vi "EventMachine.vi"() -> ()   [LabVIEW 2020]
panel:
  out "Data":i32
  in  "Events":T1
  in  "Event Data":T2
  in  "TEST":bool
  in  "INIT":bool
  in  "Stop":bool
  out "error out":errorcluster
  in  "error in":errorcluster
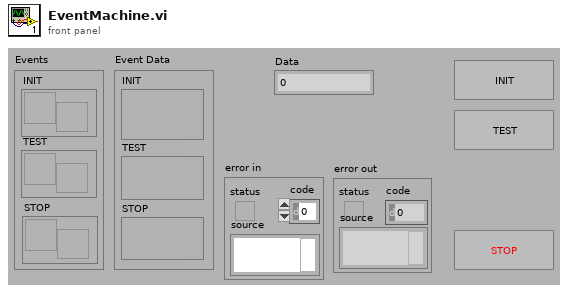
[diagram p1: front panel]
types:
  T1 = cluster{"INIT":refnum<user-event>, "TEST":refnum<user-event>, "STOP":refnum<user-event>}
  T2 = cluster{"INIT":variant, "TEST":variant, "STOP":variant}
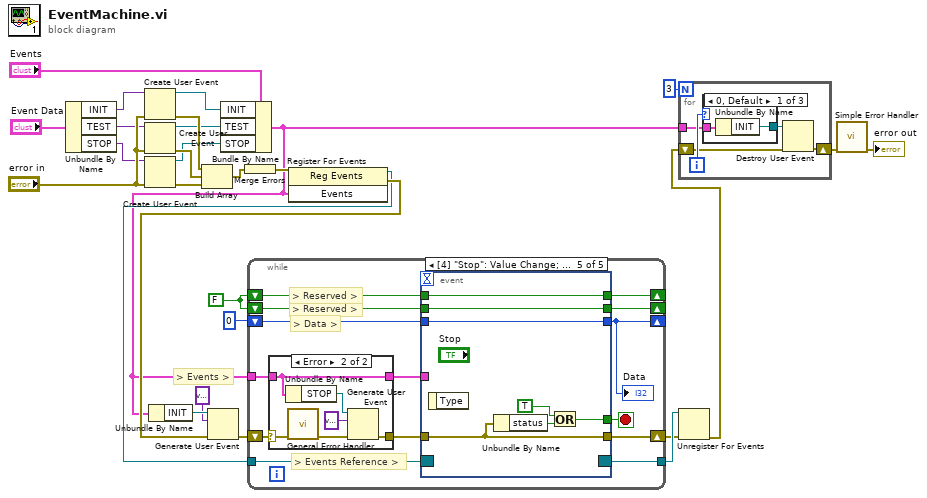
[diagram p0: block diagram]
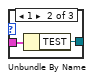
[diagram p2: hidden frame]
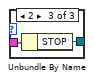
[diagram p3: hidden frame]
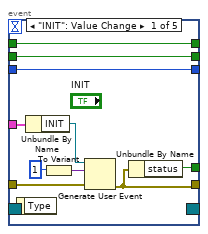
[diagram p4: hidden frame]
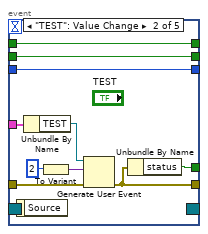
[diagram p5: hidden frame]
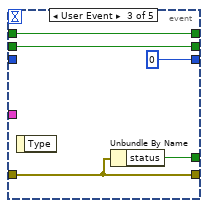
[diagram p6: hidden frame]
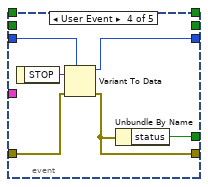
[diagram p7: hidden frame]
diagram:
  w19 = FALSE
  # "> Events >"
  n1 = Unbundle By Name("Event Data") -> ("INIT"=w12:variant, "TEST"=w11:variant, "STOP"=w6:variant)
  n2 = Create User Event(user event datatype=w12, error in="error in") -> (user event=w9:refnum<user-event>, error out=w17:errorcluster)
  n3 = Create User Event(user event datatype=w11, error in="error in") -> (user event=w8:refnum<user-event>, error out=w16:errorcluster)
  n4 = Create User Event(user event datatype=w6, error in="error in") -> (user event=w5:refnum<user-event>, error out=w3:errorcluster)
  n5 = Build Array(w17, w16, w3) -> (w15:errorcluster[])
  n6 = Bundle By Name(cluster="Events", "INIT"=w9, "TEST"=w8, "STOP"=w5) -> (w4:T1)
  n7 = Unbundle By Name(w4) -> ("INIT"=w7:refnum<user-event>)
  n8 = Merge Errors(w15) -> (w14:errorcluster)
  n9 = register-events(error in=w14, w4) -> (reference out=w25:refnum<event-registration>, error out=w27:errorcluster)  [unwired: 1 in]
  n10 = Generate User Event(user event=w7, event data cluster=variant ("event data"), error in=w27) -> (error out=w26:errorcluster)  [unwired: 1 in, 1 out]
  n11 = while {
    shift-right: [w41] -> w23
    shift-left: w26 -> [w35]
    shift-right: [w38] -> _
    shift-left: w19 -> [w36]
    shift-right: [w40] -> _
    shift-left: w19 -> [w39]
    shift-right: [w29] -> _
    shift-left: 0 -> [w37]
    tunnel: w25 -> [w33]
    tunnel: [w32] -> w24
    tunnel: w4 -> [w30]
    stop <- w42 stop-if-true
    # "> Events Reference >"
    # "> Data >"
    # "> Reserved >"
    # "> Reserved >"
    n12 = case shown="Error" w35 {
      selector: w35 -> [w82 w88]
      tunnel: [w82 w86] -> w34
      tunnel: [w81 w84] -> w31
      tunnel: w30 -> [w81 w84]
      frame No Error {
      }
      frame Error {
        n13 = Unbundle By Name(w84) -> ("STOP"=w85:refnum<user-event>)
        n14 = call <vilib>:"General Error Handler.vi"("error in (no error)"=w88) -> ("error out"=w87:errorcluster)  [unwired: 10 in, 4 out]
        n15 = Generate User Event(user event=w85, event data cluster=variant ("event data"), error in=w87) -> (error out=w86:errorcluster)  [unwired: 1 in, 1 out]
      }
    }
    n16 = event shown="[4] \"Stop\": Value Change;  <Events.STOP>: User Event" {
      selector: w33 -> [_ _ _ _ _]
      dyn-events: [_ _ _ _ _] -> w32
      timeout: _ -> [_ _ _ _ _]
      tunnel: w34 -> [w52 w62 w64 w71 w77]
      tunnel: [w51 w61 w64 w70 w77] -> w41
      tunnel: [w50 w60 w67 w73 w76] -> w42
      tunnel: w36 -> [w45 w55 w66 _ w80]
      tunnel: w39 -> [w44 w54 w65 _ w79]
      tunnel: w37 -> [w43 w53 _ w69 w78]
      tunnel: [w45 w55 w66 _ w80] -> w38
      tunnel: [w44 w54 w65 _ w79] -> w40
      tunnel: [w43 w53 0 w68 w78] -> w29
      tunnel: w31 -> [w49 w59 _ _ _]
      event "INIT": Value Change {
        n17 = event-data() -> ()  [unwired: 1 in, 1 out]
        n18 = Unbundle By Name(w49) -> ("INIT"=w48:refnum<user-event>)
        n19 = To Variant(anything=1) -> (Variant=w47:variant)
        n20 = Generate User Event(user event=w48, event data cluster=w47, error in=w52) -> (error out=w51:errorcluster)  [unwired: 1 in, 1 out]
        n21 = Unbundle By Name(w51) -> ("status"=w50:bool)
      }
      event "TEST": Value Change {
        n22 = event-data() -> ()  [unwired: 1 in, 1 out]
        n23 = Unbundle By Name(w59) -> ("TEST"=w58:refnum<user-event>)
        n24 = To Variant(anything=2) -> (Variant=w56:variant)
        n25 = Generate User Event(user event=w58, event data cluster=w56, error in=w62) -> (error out=w61:errorcluster)  [unwired: 1 in, 1 out]
        n26 = Unbundle By Name(w61) -> ("status"=w60:bool)
      }
      event User Event {
        n27 = event-data() -> ()  [unwired: 1 in, 1 out]
        n28 = Unbundle By Name(w64) -> ("status"=w67:bool)
      }
      event User Event {
        n29 = event-data() -> ("STOP"=w72:variant)  [unwired: 1 in]
        n30 = Variant To Data(error in=w71, type=w69, Variant=w72) -> (data=w68:i32, error out=w70:errorcluster)
        n31 = Unbundle By Name(w70) -> ("status"=w73:bool)
      }
      event "Stop": Value Change; User Event {
        n32 = event-data() -> ()  [unwired: 1 in, 1 out]
        n33 = Unbundle By Name(w77) -> ("status"=w74:bool)
        n34 = Or(x=TRUE ("y"), y=w74) -> (x .or. y?=w76:bool)
      }
    }
    "Data" <- w29
  }
  n35 = Unregister For Events(event registration refnum=w24, error in=w23) -> (error out=w21:errorcluster)
  n36 = for {
    N: 3 -> [_]
    shift-right: [w91] -> w20
    shift-left: w21 -> [w92]
    tunnel: w4 -> [w90]
    i -> [w93]
    n37 = case shown="0, Default" w93 {
      tunnel: [w95 w97 w99] -> w89
      tunnel: w90 -> [w94 w96 w98]
      frame 0, Default {
        n38 = Unbundle By Name(w94) -> ("INIT"=w95:refnum<user-event>)
      }
      frame 1 {
        n39 = Unbundle By Name(w96) -> ("TEST"=w97:refnum<user-event>)
      }
      frame 2 {
        n40 = Unbundle By Name(w98) -> ("STOP"=w99:refnum<user-event>)
      }
    }
    n41 = Destroy User Event ("6.销毁")(user event=w89, error in=w92) -> (error out=w91:errorcluster)
  }
  n42 = call <vilib>:"Simple Error Handler.vi"("error in (no error)"=w20) -> ("error out"=→"error out":errorcluster)  [unwired: 4 in, 4 out]
